vi "Helper SubVI - Test signal simulator.vi"() -> (3 "Test Signal":waveform(dbl))   [LabVIEW 2020]
doc: "This VI generates a sample signal for the Advanced DC-RMS Measurement.vi example."
uses:
  <vilib>/Analysis/NI_AALBase.lvlib
panel:
  # "This VI generates a sample signal for the Advanced DC-RMS Measurement.vi example."
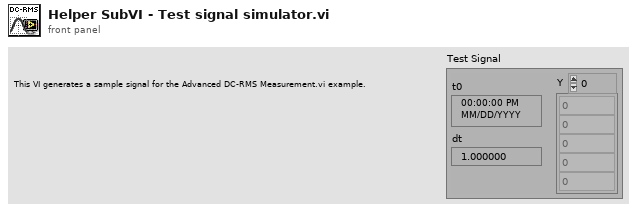
[diagram p1: front panel]
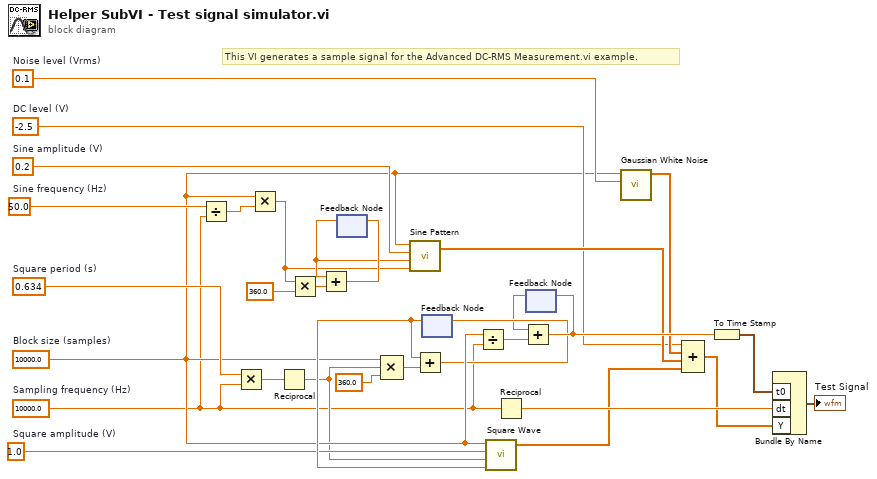
[diagram p0: block diagram]
diagram:
  w3 = 10000.0  # Sampling frequency (Hz)
  w11 = 10000.0  # Block size (samples)
  w21 = 1.0  # Square amplitude (V)
  w22 = 0.634  # Square period (s)
  w18 = 0.2  # Sine amplitude (V)
  w12 = -2.5  # DC level (V)
  w20 = 0.1  # Noise level (Vrms)
  w16 = 50.0  # Sine frequency (Hz)
  # "This VI generates a sample signal for the Advanced DC-RMS Measurement.vi example."
  n1 = Divide(x=w16, y=w3) -> (x/y=w15:dbl)
  n2 = Multiply(x=w22, y=w3) -> (x*y=w7:dbl)
  n3 = Multiply(x=w11, y=w15) -> (x*y=w14:dbl)
  n4 = Reciprocal(x=w7) -> (1/x=w5:dbl)
  n5 = Multiply(x=w14, y=360.0) -> (x*y=w13:dbl)
  n6 = feedback #1() -> (w28:dbl)  [unwired: 1 in]
  n7 = Add(x=w28, y=w13) -> (x+y=w29:dbl)
  n8 = feedback-in #1(w29) -> ()
  n9 = Compound Arithmetic op=MULTIPLY(w11, w5, 360.0) -> (w6:dbl)
  n10 = call <vilib>:"Sine Pattern.vi"("cycles"=w14, "phase(degrees)"=w28, "amplitude"=w18, "samples"=w11) -> ("Sinusoidal Pattern"=w17:dbl[])  [unwired: 1 out]
  n11 = feedback #2() -> (w27:dbl)  [unwired: 1 in]
  n12 = Add(x=w27, y=w6) -> (x+y=w10:dbl)
  n13 = feedback-in #2(w10) -> ()
  n14 = Divide(x=w11, y=w3) -> (x/y=w4:dbl)
  n15 = call <vilib>:"Square Wave.vi"("samples"=w11, "amplitude"=w21, "frequency"=w5, "phase in"=w27) -> ("square wave"=w9:dbl[])  [unwired: 2 in, 2 out]
  n16 = Reciprocal(x=w3) -> (1/x=w26:dbl)
  n17 = feedback #3() -> (w8:dbl)  [unwired: 1 in]
  n18 = Add(x=w8, y=w4) -> (x+y=w30:dbl)
  n19 = feedback-in #3(w30) -> ()
  n20 = call <vilib>:"Gaussian White Noise.vi"("standard deviation"=w20, "samples"=w11) -> ("Gaussian noise pattern"=w19:dbl[])  [unwired: 8 in, 1 out]
  n21 = Compound Arithmetic op=ADD(w12, w19, w17, w9) -> (w25:dbl[])
  n22 = To Time Stamp(1:w30) -> (0:w23:timestamp)
  n23 = Bundle By Name("t0"=w23, "dt"=w26, "Y"=w25) -> (→"Test Signal":waveform(dbl))  [unwired: 1 in]
